vi "G4BaseTemplate_Simple_4x4x4_WriteProperty.vi"(8 "error in (no error)":errorcluster, 10 "Property":dbl, 11 "reference in":refnum<class "G4BaseTemplate_Simple_4x4x4.lvclass">) -> (0 "error out":errorcluster, 3 "reference out":refnum<class "G4BaseTemplate_Simple_4x4x4.lvclass">)   [LabVIEW 2010]
uses:
  G4BaseTemplate_Simple_4x4x4.lvclass
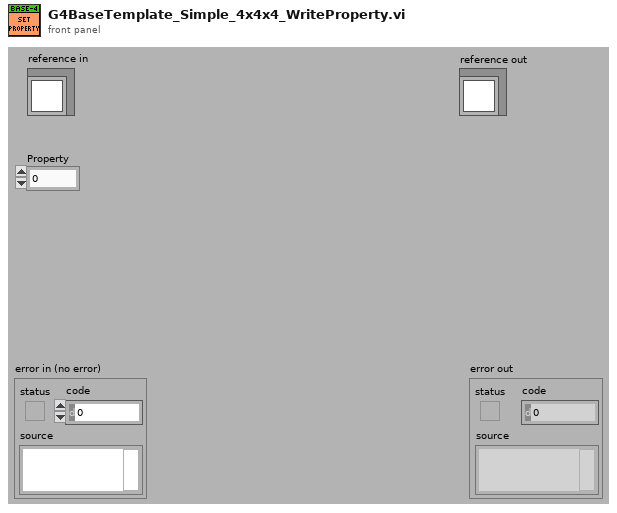
[diagram p1: front panel]
types:
  T1 = typedef "G4BaseTemplate_Simple_4x4x4.lvclass/ObjectAttributes.ctl" = cluster{"Attribute1":dbl}
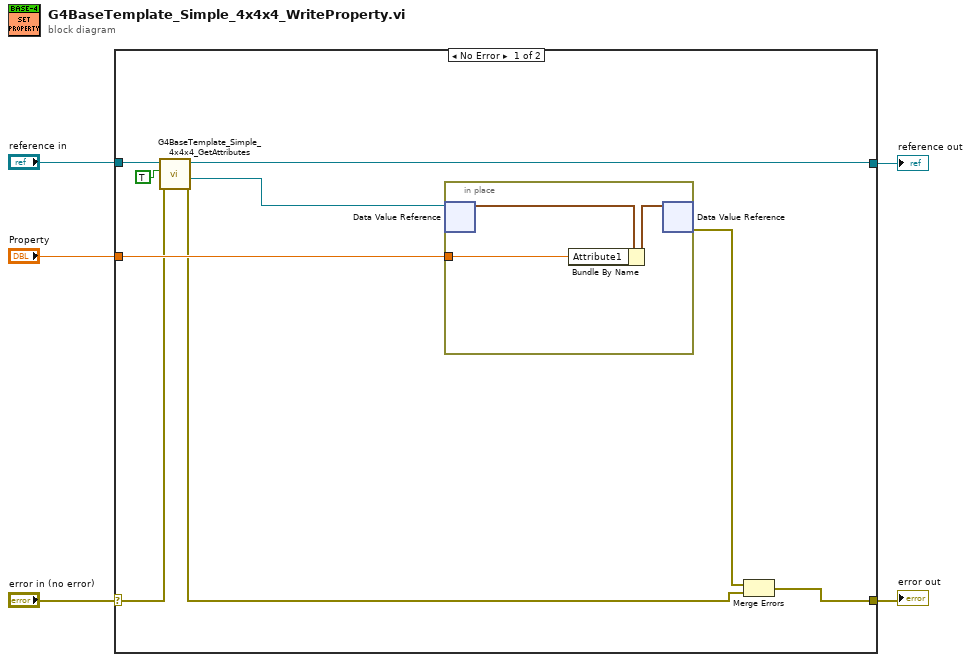
[diagram p0: block diagram]
diagram:
  n1 = case shown="No Error" "error in (no error)" {
    selector: "error in (no error)" -> [w8 w19]
    tunnel: [w12 w19] -> w4
    tunnel: [w10 w18] -> w2
    tunnel: "reference in" -> [w11 w18]
    tunnel: "Property" -> [w14 _]
    frame No Error {
      n2 = call "G4BaseTemplate_Simple_4x4x4_GetAttributes.vi"("error in (no error)"=w8, "OnlyGetDvrReference(False)"=TRUE, "reference in"=w11) -> ("error out"=w7:errorcluster, "DataRef"=w9:refnum<data-value>, "reference out"=w10:refnum<class "G4BaseTemplate_Simple_4x4x4.lvclass">)  [unwired: 5 in, 1 out]
      n3 = in-place {
        in-place-border: w14 -> [w17]
        n4 = in-place-dvr #1(w9) -> (w16:T1)  [unwired: 1 out]
        n5 = Bundle By Name(cluster=w16, "Attribute1"=w17) -> (w15:T1)
        n6 = in-place-dvr #1(w15) -> (w13:errorcluster)  [unwired: 1 out]
      }
      n7 = Merge Errors(w13, w7) -> (w12:errorcluster)
    }
    frame Error {
    }
  }
  "error out" <- w4
  "reference out" <- w2
